vi "RegisterSweepRoutedMessage_Send.vi"(8 "error in (no error)":errorcluster, 10 "RegisterSweepRoutedMessage":T1, 11 "Qbus in":refnum<class "Qbus.lvclass">) -> (0 "error out":errorcluster, 3 "Qbus out":refnum<class "Qbus.lvclass">)   [LabVIEW 2017, in "EmsaDataEventCreator.lvlib"]
uses:
  <vilib>/addons/InsightCM/Devices/Shared/Emsa/EmsaDataEventCreator/EmsaDataEventCreator.lvlib
  <vilib>/addons/Qbus/Qbus.lvclass
  <vilib>/addons/InsightCM/Devices/Shared/Emsa/EmsaDataEventCreator/controls/RegisterSweepRoutedMessage.ctl
  <vilib>/addons/InsightCM/Devices/Shared/Emsa/EmsaDataEventCreator/controls/Registry_Sweep.ctl
  <vilib>/addons/InsightCM/Devices/Shared/Common/DataEvent/controls/DataSetType.ctl
  <vilib>/addons/InsightCM/MessageBus/Base/controls/KeyValuePair.ctl
  <vilib>/addons/InsightCM/Devices/Shared/Common/DataEvent/DataEvent.lvlib
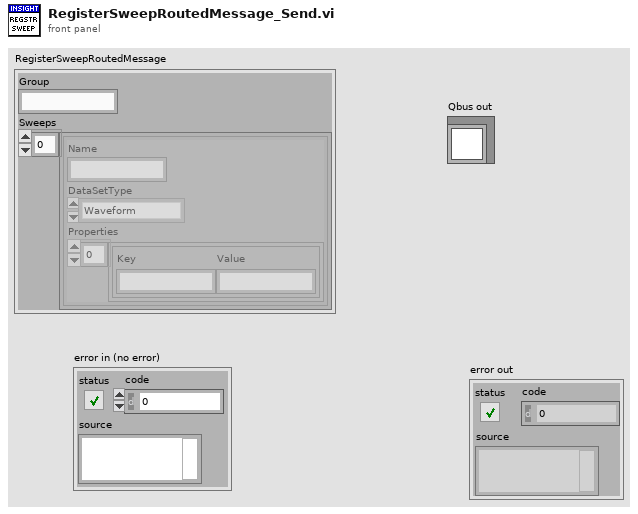
[diagram p1: front panel]
types:
  T1 = typedef "EmsaDataEventCreator.lvlib/RegisterSweepRoutedMessage.ctl" = cluster{"Group":string, "Sweeps":T2[]}
  T2 = typedef "EmsaDataEventCreator.lvlib/Registry_Sweep.ctl" = cluster{"Name":string, "DataSetType":T3, "Properties":T4[]}
  T3 = typedef "DataEvent.lvlib/DataSetType.ctl" = enum16{"Waveform", "SpeedProfile", "ThermalImage", "EmsaSweep"}
  T4 = typedef "KeyValuePair.ctl" = cluster{"Key":string, "Value":string}
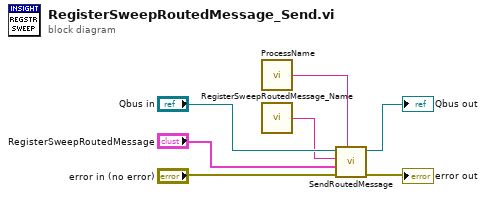
[diagram p0: block diagram]
diagram:
  n1 = call <vilib>:"ProcessName.vi"() -> ("process name"=w3:string)  [unwired: 5 in]
  n2 = call <vilib>:"RegisterSweepRoutedMessage_Name.vi"() -> ("message name"=w2:string)  [unwired: 5 in]
  n3 = call <vilib>:"SendRoutedMessage.vi"("listener process"=w3, "error in (no error)"="error in (no error)", "message value"="RegisterSweepRoutedMessage", "message name"=w2, "Qbus in"="Qbus in") -> ("error in (no error)"=→"error out":errorcluster, "Qbus out"=→"Qbus out":refnum<class "Qbus.lvclass">)  [unwired: 5 in]
